vi "Write String.vi"(8 "error in (no error)":errorcluster, 10 "Ctl Refnum":refnum<vi>, 11 "Worksheet Reference":refnum<k7>) -> (0 "error out":errorcluster)   [LabVIEW 2011, in "Design Server.lvlib"]
uses:
  Design Server.lvlib
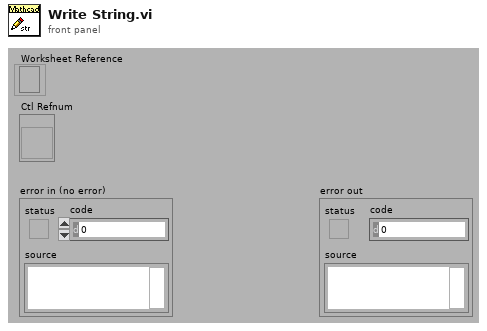
[diagram p1: front panel]
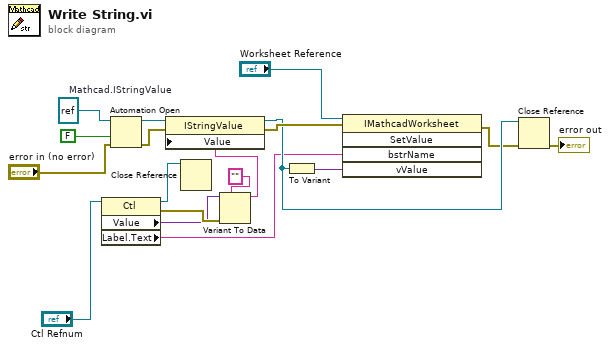
[diagram p0: block diagram]
diagram:
  w7 = refnum<k7> refnum  # Mathcad.IStringValue
  n1 = property class="Ctl"(reference="Ctl Refnum") -> (reference out=w2:refnum<vi>, error out=w10:errorcluster, "Value"=w9:variant, "Label.Text"=w11:string)  [unwired: 1 in]
  n2 = Automation Open(error in (no error)="error in (no error)", Automation Refnum=w7, 9:FALSE ("open new instance")) -> (Automation Refnum=w17:refnum<k7>, error out=w16:errorcluster)  [unwired: 1 in]
  n3 = Close Reference(reference=w2) -> ()  [unwired: 1 in, 1 out]
  n4 = Variant To Data(error in=w10, type="", Variant=w9) -> (data=w8:string)  [unwired: 1 out]
  n5 = property class="IStringValue"(reference=w17, error in=w16, "Value"=w8) -> (reference out=w13:refnum<k7>, error out=w14:errorcluster)
  n6 = To Variant(anything=w13) -> (Variant=w15:variant)
  n7 = invoke class="IMathcadWorksheet" method="SetValue"(reference="Worksheet Reference", error in=w14, "bstrName"=w11, "vValue"=w15) -> (error out=w12:errorcluster)  [unwired: 1 in, 4 out]
  n8 = Close Reference(reference=w13, error in (no error)=w12) -> (error out=→"error out":errorcluster)
